vi "Log Trace.vi"(8 "error in (no error)":errorcluster, 10 "Trace.lvclass":refnum<class "Trace.lvclass">, 11 "Tracer-P in":refnum<class "Tracer-P.lvclass">) -> (0 "error out":errorcluster, 2 "TraceMessage Out":refnum<class "Trace.lvclass">, 3 "Tracer-P out":refnum<class "Tracer-P.lvclass">)   [LabVIEW 2013, in "Tracer-P.lvclass"]
uses:
  Tracer-P.lvclass
  Logical Systems/TraceMessage/Trace.lvclass
  Logical Systems/Tracer/Tracer.lvclass
  Tracer-P.lvclass/Tracer-P.ctl
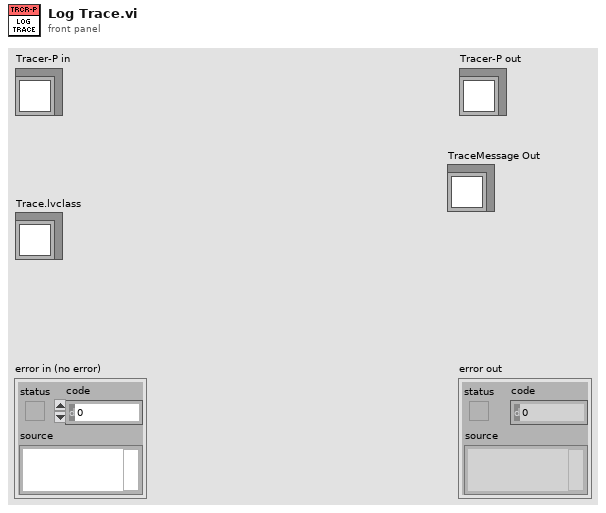
[diagram p1: front panel]
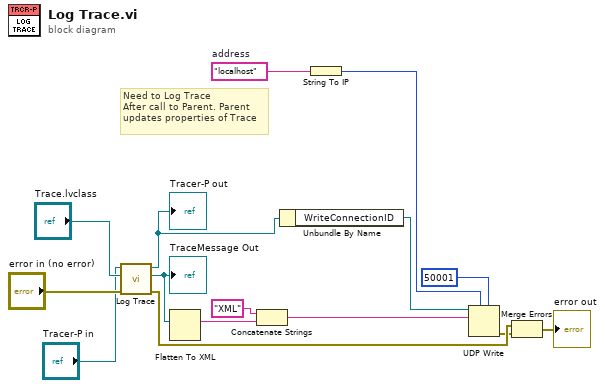
[diagram p0: block diagram]
diagram:
  w10 = "localhost"  # address
  # "Need to Log Trace\nAfter call to Parent. Parent\nupdates properties of Trace"
  n1 = call-parent "Log Trace.vi"("error in (no error)"="error in (no error)", "Trace.lvclass"="Trace.lvclass", "Tracer in"="Tracer-P in") -> ("error out"=w2:errorcluster, "TraceMessage Out"=w6:refnum<class "Trace.lvclass">, "Tracer out"=w12:refnum<class "Tracer-P.lvclass">)  [unwired: 6 in]
  "Tracer-P out" <- w12
  "TraceMessage Out" <- w6
  n2 = Flatten To XML(anything=w6) -> (xml string=w5:string)
  n3 = Concatenate Strings("XML" ("string"), w5) -> (w8:string)
  n4 = Unbundle By Name(w12) -> ("WriteConnectionID"=w11:refnum<k16>)
  n5 = String To IP(1:w10) -> (0:w9:u32)
  n6 = UDP Write(address=w9, port or service name=u16 50001, connection ID=w11, data in=w8) -> (error out=w1:errorcluster)  [unwired: 2 in, 1 out]
  n7 = Merge Errors(w2, w1) -> (→"error out":errorcluster)
